vi "VGI Write Datas.vi"(7 "Data":u16, 8 "error in (no error)":errorcluster, 9 "PinMask":u16, 10 "DevIndex":i32, 11 "DevType":i32) -> (0 "error out":errorcluster, 3 "function return":i32)   [LabVIEW 2012, in "ControlGPIO.lvlib"]
doc: "int WINAPI VGI_WriteDatas(int DevType,int DevIndex, unsigned short PinMask,unsigned short Data);"
uses:
  ControlGPIO.lvlib
  Ginkgo_Driver.dll
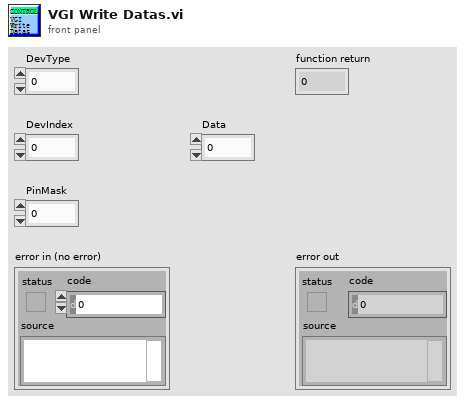
[diagram p1: front panel]
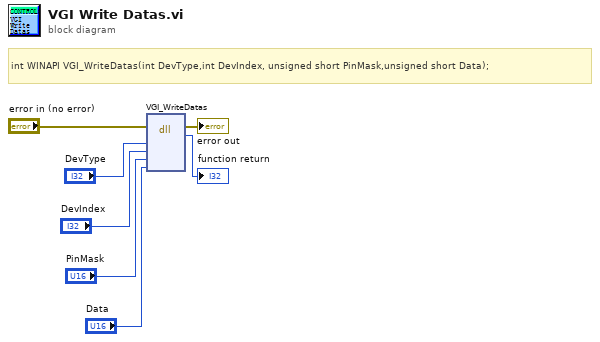
[diagram p0: block diagram]
diagram:
  # "int WINAPI VGI_WriteDatas(int DevType,int DevIndex, unsigned short PinMask,unsigned short Data);"
  n1 = dll-call lib="E:/Project/vt_ginkgo/truck/Ginkgo Driver/vs2010/Ginkgo_USB-I2C_API_v2.0.3.0/lib/labview_32bit/ControlGPIO/Ginkgo_Driver.*" fn="VGI_WriteDatas"(error in="error in (no error)", "DevType"="DevType", "DevIndex"="DevIndex", "PinMask"="PinMask", "Data"="Data") -> (error out=→"error out":errorcluster, →"function return":i32)  [unwired: 6 in, 1 out]
